vi "Write Config. Data.vi"(8 "error in (no error)":errorcluster, 10 "Config. Data":T1, 11 "Template Action Cfg in":refnum<class "Template Action Cfg.lvclass">) -> (0 "error out":errorcluster, 3 "Template Action Cfg out":refnum<class "Template Action Cfg.lvclass">)   [LabVIEW 2014, in "Template Action Cfg.lvclass"]
uses:
  Template Action Cfg.lvclass
  configuration data.ctl
  Template Action Cfg.lvclass/Template Action Cfg.ctl
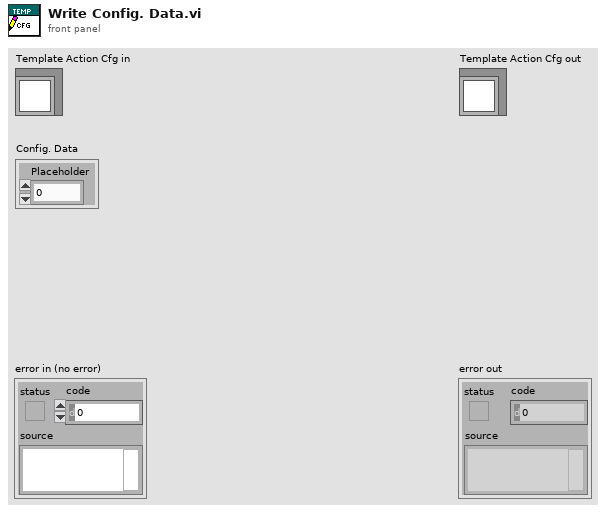
[diagram p1: front panel]
types:
  T1 = typedef "Template Action Cfg.lvclass/configuration data.ctl" = cluster{"Placeholder":dbl}
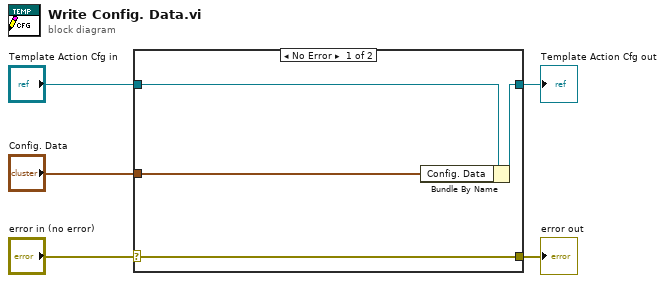
[diagram p0: block diagram]
diagram:
  n1 = case shown="No Error" "error in (no error)" {
    selector: "error in (no error)" -> [w9 w10]
    tunnel: [w9 w10] -> w4
    tunnel: [w7 w11] -> w2
    tunnel: "Template Action Cfg in" -> [w8 w11]
    tunnel: "Config. Data" -> [w6 _]
    frame No Error {
      n2 = Bundle By Name(cluster=w8, "Config. Data"=w6) -> (w7:refnum<class "Template Action Cfg.lvclass">)
    }
    frame Error {
    }
  }
  "error out" <- w4
  "Template Action Cfg out" <- w2
